vi "Constructor_EventLogHandle.vi"(8 "error in (no error)":errorcluster) -> (0 "error out":errorcluster, 3 "EventHandle":refnum<class "EventLogHandle.lvclass">)   [LabVIEW 2024, in "EventLogHandle.lvclass"]
uses:
  EventLogHandle.lvclass
  EventLogHandle.lvclass/EventLogHandle.ctl
  Record/LogRecord.lvclass
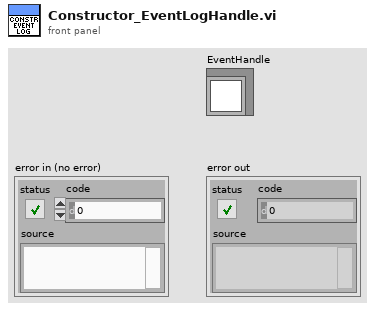
[diagram p1: front panel]
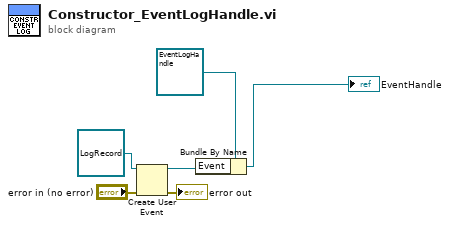
[diagram p0: block diagram]
diagram:
  n1 = Create User Event(user event datatype=refnum<class "LogRecord.lvclass"> refnum ("LogRecord.lvclass"), error in="error in (no error)") -> (user event=w5:refnum<user-event>, error out=→"error out":errorcluster)
  n2 = Bundle By Name(cluster=refnum<class "EventLogHandle.lvclass"> refnum ("EventLogHandle.lvclass"), "Event"=w5) -> (→"EventHandle":refnum<class "EventLogHandle.lvclass">)
